vi "Initialize.vi"(6 "TCS COM Port":string="COM1", 7 "Remote IP":string="200.131.64.49", 8 "error in (no error)":errorcluster, 9 "TCS Simulated/Real":bool, 10 "channels quantity":i32, 11 "SPARC4_GUI in":refnum<class "SPARC4_GEI.lvclass">) -> (0 "error out":errorcluster, 3 "SPARC4_GUI out":refnum<class "SPARC4_GEI.lvclass">)   [LabVIEW 2018, in "SPARC4_GEI.lvclass"]
uses:
  SPARC4_GEI.lvclass
  Channel GUI/Channel GEI.lvclass
  Channel GUI/Channel GEI.lvclass/Channel GEI.ctl
  SPARC4_GEI.lvclass/SPARC4_GEI.ctl
  Filter_Wheel/Filter_Wheel.lvclass
panel:
  in  "Channel GUI.lvclass":refnum<class "Channel GEI.lvclass">
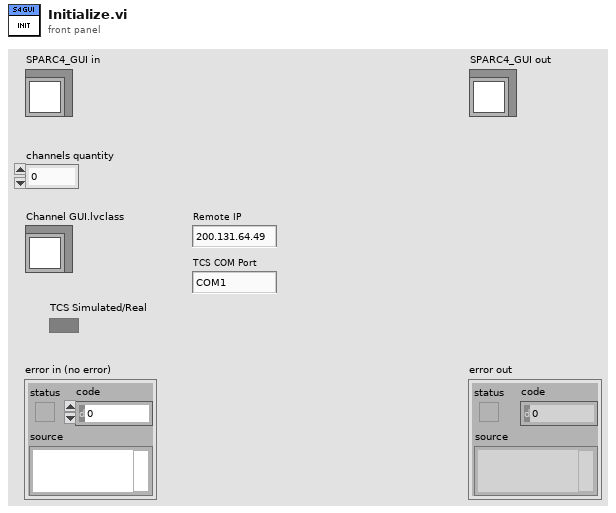
[diagram p1: front panel]
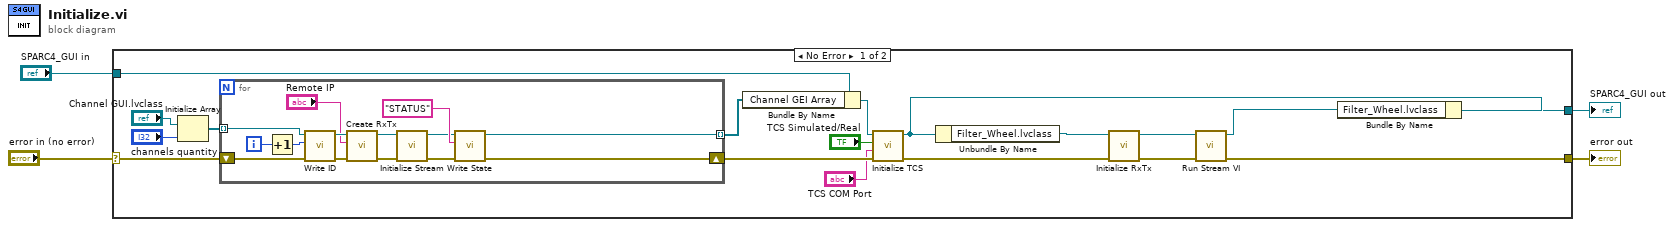
[diagram p0: block diagram]
diagram:
  n1 = case shown="No Error" "error in (no error)" {
    selector: "error in (no error)" -> [w20 w38]
    tunnel: [w7 w38] -> w3
    tunnel: [w6 w37] -> w1
    tunnel: "SPARC4_GUI in" -> [w18 w37]
    frame No Error {
      n2 = Initialize Array("Channel GUI.lvclass", "channels quantity") -> (w21:refnum<class "Channel GEI.lvclass">[])
      n3 = for {
        shift-right: [w28] -> w16
        shift-left: w20 -> [w35]
        tunnel: w21 -> [w36] mode=indexing
        tunnel: [w27] -> w19 mode=indexing
        i -> [w31]
        n4 = Increment(x=w31) -> (x+1=w32:i32)
        n5 = call "Write ID.vi"("error in (no error)"=w35, "ID"=w32, "Channel GUI in"=w36) -> ("error out"=w34:errorcluster, "Channel GUI out"=w33:refnum<class "Channel GEI.lvclass">)  [unwired: 7 in]
        n6 = call "Create RxTx.vi"("error in (no error)"=w34, "Remote IP"="Remote IP", "Channel GUI in"=w33) -> ("error out"=w29:errorcluster, "Channel GUI out"=w30:refnum<class "Channel GEI.lvclass">)  [unwired: 7 in]
        n7 = call "Initialize Stream.vi"("error in (no error)"=w29, "Channel GUI in"=w30) -> ("error out"=w24:errorcluster, "Channel GUI out"=w25:refnum<class "Channel GEI.lvclass">)  [unwired: 8 in]
        n8 = call "Write State.vi"("error in (no error)"=w24, "State"="STATUS", "Channel GEI in"=w25) -> ("error out"=w28:errorcluster, "Channel GEI out"=w27:refnum<class "Channel GEI.lvclass">)  [unwired: 7 in]
      }
      n9 = Bundle By Name(cluster=w18, "Channel GEI Array"=w19) -> (w17:refnum<class "SPARC4_GEI.lvclass">)
      n10 = call "Initialize TCS.vi"("error in (no error)"=w16, "TCS COM Port"="TCS COM Port", "TCS Simulated/Real"="TCS Simulated/Real", "SPARC4_GEI in"=w17) -> ("error out"=w12:errorcluster, "SPARC4_GEI out"=w9:refnum<class "SPARC4_GEI.lvclass">)  [unwired: 6 in]
      n11 = Unbundle By Name(w9) -> ("Filter_Wheel.lvclass"=w13:refnum<class "Filter_Wheel.lvclass">)
      n12 = call "Initialize RxTx.vi"("error in (no error)"=w12, "Filter_Wheel in"=w13) -> ("error out"=w11:errorcluster, "Filter_Wheel out"=w10:refnum<class "Filter_Wheel.lvclass">)  [unwired: 8 in]
      n13 = call "Run Stream VI.vi"("error in (no error)"=w11, "Filter_Wheel in"=w10) -> ("error out"=w7:errorcluster, "Filter_Wheel out"=w8:refnum<class "Filter_Wheel.lvclass">)  [unwired: 8 in]
      n14 = Bundle By Name(cluster=w9, "Filter_Wheel.lvclass"=w8) -> (w6:refnum<class "SPARC4_GEI.lvclass">)
    }
    frame Error {
    }
  }
  "error out" <- w3
  "SPARC4_GUI out" <- w1
